vi "Get Mac Address.vi"() -> (1 "MAC Address":string)   [LabVIEW 2015]
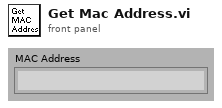
[diagram p1: front panel]
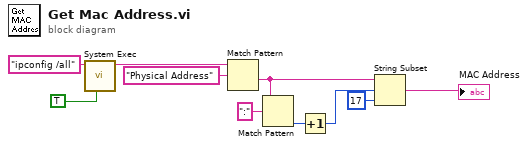
[diagram p0: block diagram]
diagram:
  n1 = call <vilib>:"System Exec.vi"("run minimized? (F)"=TRUE, "command line"="ipconfig /all") -> ("standard output"=w8:string)  [unwired: 6 in, 3 out]
  n2 = Match Pattern(string=w8, regular expression="Physical Address") -> (after substring=w5:string)  [unwired: 1 in, 3 out]
  n3 = Match Pattern(string=w5, regular expression=":") -> (offset past match=w4:i32)  [unwired: 1 in, 3 out]
  n4 = Increment(x=w4) -> (x+1=w2:i32)
  n5 = String Subset(string=w5, offset (0)=w2, length (rest)=17 ("length (rest)")) -> (substring=→"MAC Address":string)
